vi "set debug write.vi"(8 "error in (no error)":errorcluster, 10 "debug_write":T1, 11 "id":i32) -> (0 "error out":errorcluster, 3 "function return":i32)   [LabVIEW 2012, in "libximc.lvlib"]
doc: "result_t XIMC_API set_debug_write (device_t id, const debug_write_t* debug_write);"
uses:
  libximc.lvlib
  libximc.dll
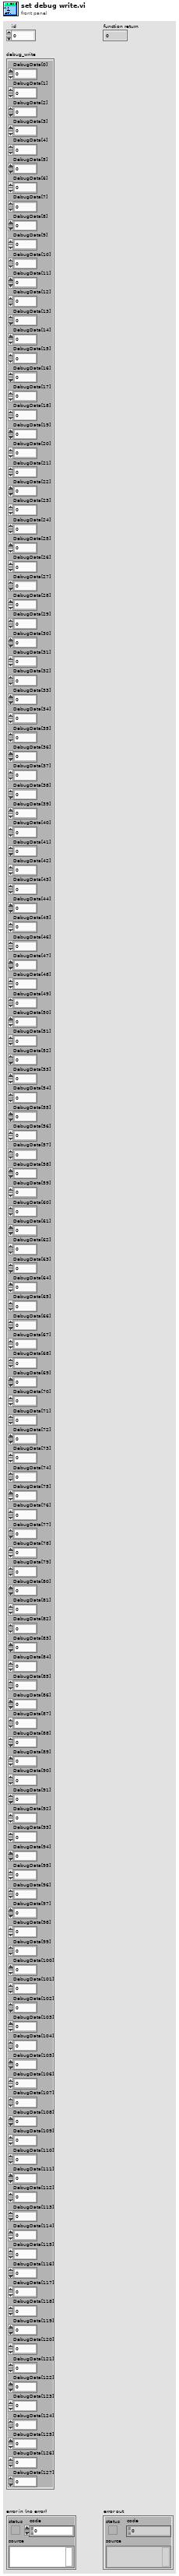
[diagram p1: front panel]
types:
  T1 = cluster{"DebugData[0]":u8, "DebugData[1]":u8, "DebugData[2]":u8, "DebugData[3]":u8, "DebugData[4]":u8, "DebugData[5]":u8, "DebugData[6]":u8, "DebugData[7]":u8, "DebugData[8]":u8, "DebugData[9]":u8, "DebugData[10]":u8, "DebugData[11]":u8, "DebugData[12]":u8, "DebugData[13]":u8, "DebugData[14]":u8, "DebugData[15]":u8, "DebugData[16]":u8, "DebugData[17]":u8, "DebugData[18]":u8, "DebugData[19]":u8, "DebugData[20]":u8, "DebugData[21]":u8, "DebugData[22]":u8, "DebugData[23]":u8, "DebugData[24]":u8, "DebugData[25]":u8, "DebugData[26]":u8, "DebugData[27]":u8, "DebugData[28]":u8, "DebugData[29]":u8, "DebugData[30]":u8, "DebugData[31]":u8, "DebugData[32]":u8, "DebugData[33]":u8, "DebugData[34]":u8, "DebugData[35]":u8, "DebugData[36]":u8, "DebugData[37]":u8, "DebugData[38]":u8, "DebugData[39]":u8, "DebugData[40]":u8, "DebugData[41]":u8, "DebugData[42]":u8, "DebugData[43]":u8, "DebugData[44]":u8, "DebugData[45]":u8, "DebugData[46]":u8, "DebugData[47]":u8, "DebugData[48]":u8, "DebugData[49]":u8, "DebugData[50]":u8, "DebugData[51]":u8, "DebugData[52]":u8, "DebugData[53]":u8, "DebugData[54]":u8, "DebugData[55]":u8, "DebugData[56]":u8, "DebugData[57]":u8, "DebugData[58]":u8, "DebugData[59]":u8, "DebugData[60]":u8, "DebugData[61]":u8, "DebugData[62]":u8, "DebugData[63]":u8, "DebugData[64]":u8, "DebugData[65]":u8, "DebugData[66]":u8, "DebugData[67]":u8, "DebugData[68]":u8, "DebugData[69]":u8, "DebugData[70]":u8, "DebugData[71]":u8, "DebugData[72]":u8, "DebugData[73]":u8, "DebugData[74]":u8, "DebugData[75]":u8, "DebugData[76]":u8, "DebugData[77]":u8, "DebugData[78]":u8, "DebugData[79]":u8, "DebugData[80]":u8, "DebugData[81]":u8, "DebugData[82]":u8, "DebugData[83]":u8, "DebugData[84]":u8, "DebugData[85]":u8, "DebugData[86]":u8, "DebugData[87]":u8, "DebugData[88]":u8, "DebugData[89]":u8, "DebugData[90]":u8, "DebugData[91]":u8, "DebugData[92]":u8, "DebugData[93]":u8, "DebugData[94]":u8, "DebugData[95]":u8, "DebugData[96]":u8, "DebugData[97]":u8, "DebugData[98]":u8, "DebugData[99]":u8, "DebugData[100]":u8, "DebugData[101]":u8, "DebugData[102]":u8, "DebugData[103]":u8, "DebugData[104]":u8, "DebugData[105]":u8, "DebugData[106]":u8, "DebugData[107]":u8, "DebugData[108]":u8, "DebugData[109]":u8, "DebugData[110]":u8, "DebugData[111]":u8, "DebugData[112]":u8, "DebugData[113]":u8, "DebugData[114]":u8, "DebugData[115]":u8, "DebugData[116]":u8, "DebugData[117]":u8, "DebugData[118]":u8, "DebugData[119]":u8, "DebugData[120]":u8, "DebugData[121]":u8, "DebugData[122]":u8, "DebugData[123]":u8, "DebugData[124]":u8, "DebugData[125]":u8, "DebugData[126]":u8, "DebugData[127]":u8}
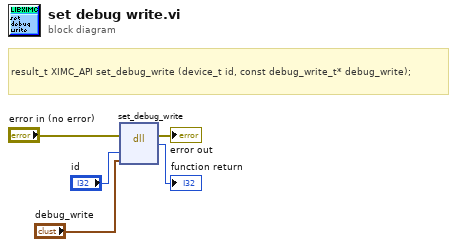
[diagram p0: block diagram]
diagram:
  # "result_t XIMC_API set_debug_write (device_t id, const debug_write_t* debug_write);"
  n1 = dll-call lib="C:/Users/Stepan/Downloads/labview_2.9.11_testgen_thread/libximc.*" fn="set_debug_write"(error in="error in (no error)", "id"="id", "debug_write"="debug_write") -> (error out=→"error out":errorcluster, →"function return":i32)  [unwired: 4 in, 1 out]
